vi "Server Print Test.vi"() -> ()   [LabVIEW 2014, in "ESP8266 WiFi Wrapper.lvlib"]
uses:
  <vilib>/Aledyne-TSXperts/Arduino Compatible Compiler for LabVIEW/addons/ESP8266 WiFi Wrapper/ESP8266 WiFi Wrapper.lvlib
panel:
  out "Bytes written":u16
  in  "String to write":string
  out "Error Out":errorcluster
  in  "Error In":errorcluster
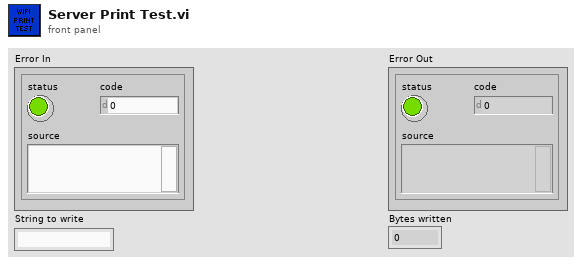
[diagram p1: front panel]
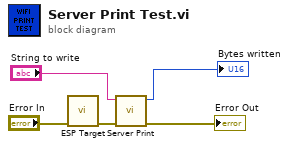
[diagram p0: block diagram]
diagram:
  n1 = call <vilib>:"ESP Target.vi"("Error In"="Error In") -> ("Error Out"=w1:errorcluster)  [unwired: 10 in]
  n2 = call <vilib>:"Server Print.vi"("Error In"=w1, "String to write"="String to write") -> ("Error Out"=→"Error Out":errorcluster, "Bytes written"=→"Bytes written":u16)  [unwired: 8 in]
